vi "AvoidTypeZeroOrLesser.vi"(10 "User Input":string, 11 "data in":string) -> (1 "Boolean":bool, 2 "Numeric":i32, 3 "Numeric 2":i32)   [LabVIEW 2020]
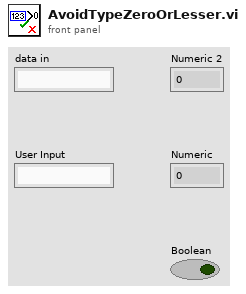
[diagram p1: front panel]
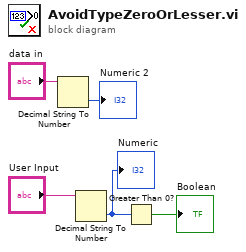
[diagram p0: block diagram]
diagram:
  n1 = Decimal String To Number(string="data in") -> (number=→"Numeric 2":i32)  [unwired: 2 in, 1 out]
  n2 = Decimal String To Number(string="User Input") -> (number=w5:i32)  [unwired: 2 in, 1 out]
  "Numeric" <- w5
  n3 = Greater Than 0?(x=w5) -> (x > 0?=→"Boolean":bool)
